vi "HumanSelectDriveMode_OLD.vi"(4 "AutoTrajStageLeft":bool, 5 "AutoTrajSource":bool, 6 "AutoTrajStageCenter":bool, 7 "AutoTrajAmp":bool, 8 "AutoTrajSpeakerRight":bool, 9 "AutoTrajSpeakerCenter":bool, 10 "AutoTrajStageRight":bool, 11 "FollowButtonTraj":bool) -> (3 "Drive Mode":i32)   [LabVIEW 2023]
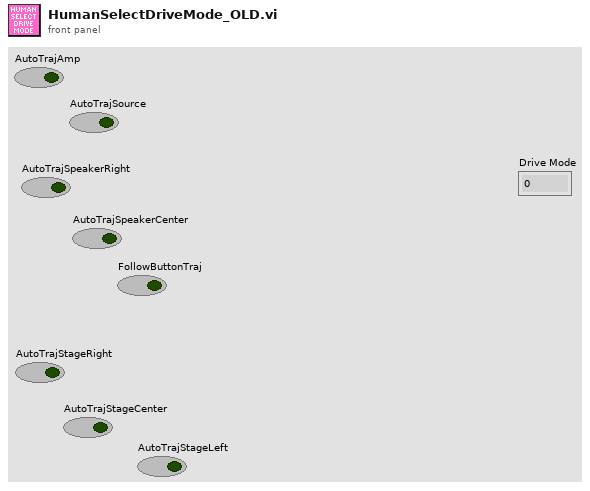
[diagram p1: front panel]
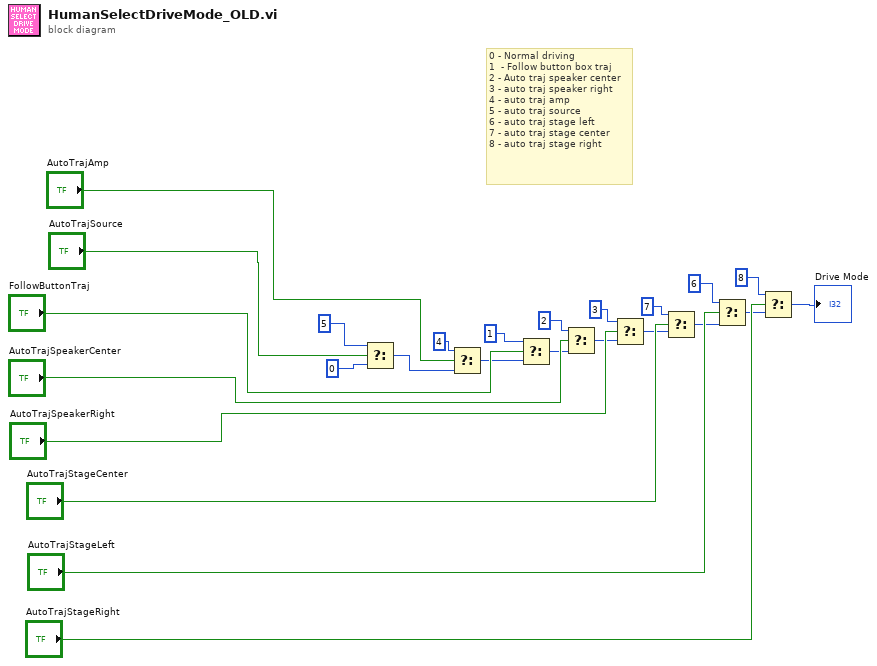
[diagram p0: block diagram]
diagram:
  # "0 - Normal driving\n1  - Follow button box traj\n2 - Auto traj speaker center\n3 - auto traj speaker right \n4 - auto traj amp\n5 - auto traj source\n6 - auto traj stage left\n7 - auto traj stage center\n8 - auto traj stage right"
  n1 = Select(t=5, s="AutoTrajSource", f=0) -> (s? t:f=w5:i32)
  n2 = Select(t=4, s="AutoTrajAmp", f=w5) -> (s? t:f=w6:i32)
  n3 = Select(t=1, s="FollowButtonTraj", f=w6) -> (s? t:f=w7:i32)
  n4 = Select(t=2, s="AutoTrajSpeakerCenter", f=w7) -> (s? t:f=w8:i32)
  n5 = Select(t=3, s="AutoTrajSpeakerRight", f=w8) -> (s? t:f=w9:i32)
  n6 = Select(t=7, s="AutoTrajStageCenter", f=w9) -> (s? t:f=w10:i32)
  n7 = Select(t=6, s="AutoTrajStageLeft", f=w10) -> (s? t:f=w11:i32)
  n8 = Select(t=8, s="AutoTrajStageRight", f=w11) -> (s? t:f=→"Drive Mode":i32)
